vi "Unflatten DataCNT to DVR.vi"(1 "Data Contianer":T2) -> (0 "DataCNT DVR":T1)   [LabVIEW 2017, in "Data Container.lvlib"]
uses:
  Data Container.lvlib
  TypeDef/Def-DataCNT.ctl
  TypeDef/Def-DataCNT Ico.ctl
  TypeDef/Def-DataCNT DVR.ctl
panel:
  # "Connector Pane"
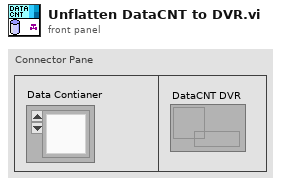
[diagram p1: front panel]
types:
  T1 = typedef "Data Container.lvlib/Def-DataCNT DVR.ctl" = refnum<data-value>
  T2 = typedef "Data Container.lvlib/Def-DataCNT.ctl" = refnum<k1>
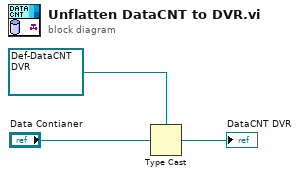
[diagram p0: block diagram]
diagram:
  n1 = Type Cast(type=T1 refnum ("DataCNT Reference"), x="Data Contianer") -> (*(type *) &x=→"DataCNT DVR":T1)
